vi "Sub Initialize.vi"(6 "Controller name":string, 8 "error in (no error)":errorcluster, 11 "Spectrum Recorder in":refnum<class "Spectrum Recorder too.lvclass">) -> (0 "error out":errorcluster, 2 "Initialize Result":refnum<class "Acquired Result.lvclass">, 3 "Spectrum Recorder out":refnum<class "Spectrum Recorder too.lvclass">)   [LabVIEW 2024, in "Spectrum Recorder too.lvclass"]
uses:
  Spectrum Recorder too.lvclass
  NHMFL_Core/Libraries/Instruments/Results/Acquired Result/Acquired Result.lvclass
  Worker/Worker Actor/Worker Actor.lvclass/Worker Actor.ctl
  Spectrum Recorder too.lvclass/Spectrum Recorder too.ctl
  Publish-Subscribe/Context.ctl
  <vilib>/ActorFramework/Actor/Actor.lvclass/Actor.ctl
  <vilib>/ActorFramework/Message Enqueuer/Message Enqueuer.lvclass/Message Enqueuer.ctl
  Publish-Subscribe/Interfaces/Publisher Messages/Subscribe Msg/Subscribe Msg.lvclass/Subscribe Msg.ctl
  NHMFL_Core/Libraries/Instruments/Instrument Driver/Worker State.ctl
  Write Fine region centers.vi
  Template Module/Write State.vi
  Template Module/Read State.vi
  <vilib>/ActorFramework/Message Enqueuer/Init from Existing Queue.vi
  <vilib>/ActorFramework/Message Enqueuer/Enqueue.vi
  Publish-Subscribe/Interfaces/Publisher Messages/Subscribe Msg/Subscribe Msg.lvclass
  Read Spectrum Recorder Configuration.vi
  <vilib>/ActorFramework/Message Priority Queue/Priority Enqueue.vi
  <vilib>/ActorFramework/Message Enqueuer/Message Enqueuer.lvclass
  Recorders/Continuous Recorder Actor/Continuous Recorder Actor.lvclass
  <vilib>/ActorFramework/Actor/Actor.lvclass
  D:/GitHub/LabActor/Recorders/Continuous Recorder Actor/Continuous Recorder Actor.lvclass
  D:/GitHub/LabActor/Instrument Actor/Instrument Actor.lvclass
  D:/GitHub/LabActor/Worker/Worker Actor/Worker Actor.lvclass
  D:/GitHub/LabActor/Template Module/Template Module.lvclass
  C:/Program Files/National Instruments/LabVIEW 2024/vi.lib/ActorFramework/Actor/Actor.lvclass
  D:/GitHub/LabActor/Worker/Woker Interface/Worker.lvclass
  D:/GitHub/LabActor/Recorders/Interfaces/Continuous Recorder/Continuous Recorder.lvclass
  D:/GitHub/LabActor/Spectrum Recorder too/Spectrum Recorder too.lvclass
  D:/GitHub/LabActor/Publish-Subscribe/Interfaces/Subscriber/Subscriber.lvclass
  NHMFL_Core/Libraries/Red Pitaya/RP Core/RP Transceiver/RP Transceiver.lvclass
  NHMFL_Core/Libraries/Red Pitaya/RP Core/RP Transceiver/Receiver format.ctl
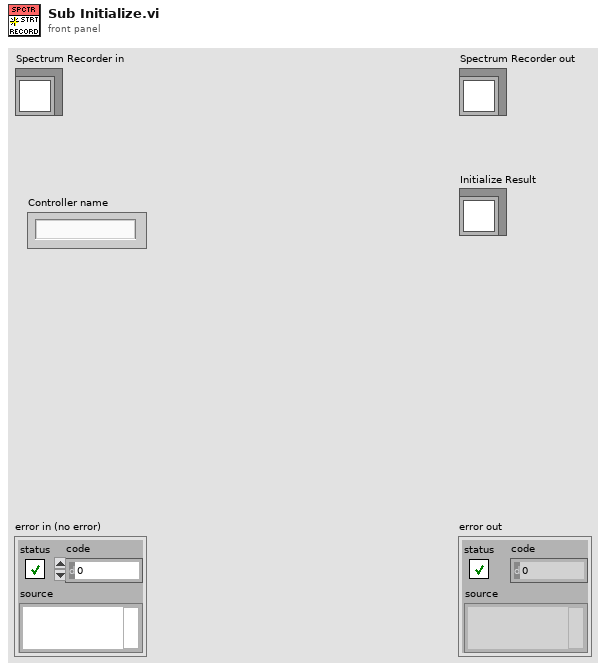
[diagram p1: front panel]
types:
  T1 = typedef "Receiver format.ctl" = enum16{"Hub 2xy", "Hub port 2xy 4f", "Hub ports 234", "X-Y-F", "F-X-Y", "X-Y", "X"}
  T2 = typedef "Context.ctl" = cluster{"Topic":string, "Source":string}
  T3 = typedef "Worker State.ctl" = enum16{"Idle", "Starting", "Working", "Stopping"}
  T4 = typedef "Spectrum Configuration.ctl" = cluster{"Start frequency":dbl, "End frequency":dbl, "Coarse step":dbl, "Step duration":dbl, "Red Pitaya address":string, "Open plot \non start":bool, "Regions width":dbl, "Fine step":dbl, "Pause between scans":dbl, "Clear rgs on start":bool, "Output amplitude":dbl, "Append measurements":string[], "Full scan period":dbl, "Full start":dbl, "Full end":dbl, "Full step":dbl}
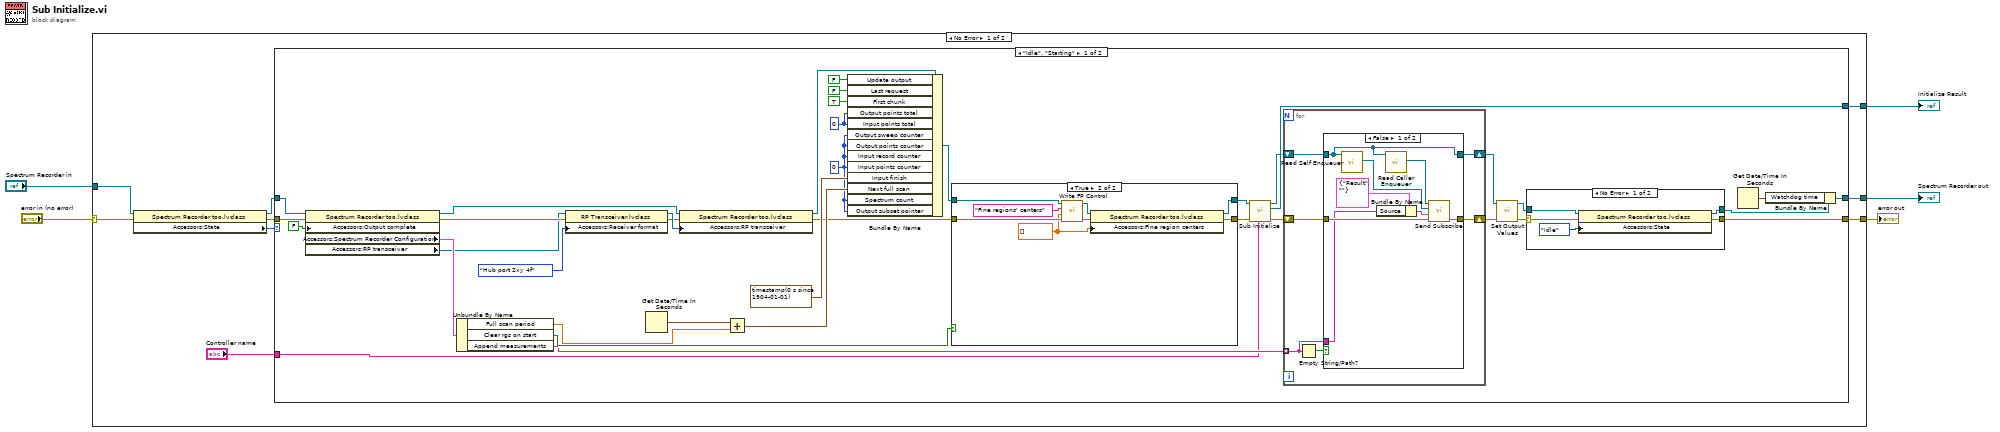
[diagram p0: block diagram]
diagram:
  n1 = case shown="No Error" "error in (no error)" {
    selector: "error in (no error)" -> [w9 w89]
    tunnel: [w12 w89] -> w4
    tunnel: [w14 w88] -> w2
    tunnel: "Spectrum Recorder in" -> [w13 w88]
    tunnel: [w7 _] -> w1
    frame No Error {
      n2 = property class="Spectrum Recorder too.lvclass"(reference=w13, error in=w9) -> (reference out=w11:refnum<class "Spectrum Recorder too.lvclass">, error out=w8:errorcluster, "Accessors:State"=w10:T3)
      n3 = case shown="\"Idle\", \"Starting\"" w10 {
        tunnel: w11 -> [w46 w87]
        tunnel: [w29 w87] -> w14
        tunnel: w8 -> [w45 w86]
        tunnel: [w52 w86] -> w12
        tunnel: [w43 _] -> w7
        tunnel: "Controller name" -> [w27 _]
        frame "Idle", "Starting" {
          w47 = i64 0 ("Output points total")
          w23 = 0 ("Output sweep counter")
          n4 = property class="Spectrum Recorder too.lvclass"(reference=w46, error in=w45, "Accessors:Output complete"=FALSE ("Output complete")) -> (reference out=w22:refnum<class "Spectrum Recorder too.lvclass">, error out=w20:errorcluster, "Accessors:Spectrum Recorder Configuration"=w40:T4, "Accessors:RP transceiver"=w19:refnum<class "RP Transceiver.lvclass">)
          n5 = Unbundle By Name(w40) -> ("Full scan period"=w25:dbl, "Clear rgs on start"=w39:bool, "Append measurements"=w34:string[])
          n6 = property class="RP Transceiver.lvclass"(reference=w19, error in=w20, "Accessors:Receiver format"=Receiver_format."Hub port 2xy 4f" ("Receiver format")) -> (reference out=w18:refnum<class "RP Transceiver.lvclass">, error out=w16:errorcluster)
          n7 = Get Date/Time In Seconds() -> (seconds since 1Jan1904=w26:timestamp)
          n8 = property class="Spectrum Recorder too.lvclass"(reference=w22, error in=w16, "Accessors:RP transceiver"=w18) -> (reference out=w17:refnum<class "Spectrum Recorder too.lvclass">, error out=w15:errorcluster)
          n9 = Add(x=w26, y=w25) -> (x+y=w24:timestamp)
          n10 = Bundle By Name(cluster=w17, "Update output"=FALSE, "Last request"=FALSE, "First chunk"=TRUE, "Output points total"=w47, "Input points total"=w47, "Output sweep counter"=w23, "Output points counter"=w23, "Input record counter"=w23, "Input points counter"=w23, "Input finish"=timestamp(0 s since 1904-01-01), "Next full scan"=w24, "Spectrum count"=w23, "Output subset pointer"=w23) -> (w38:refnum<class "Spectrum Recorder too.lvclass">)
          n11 = case shown="True" w39 {
            tunnel: w38 -> [w70 w78]
            tunnel: w15 -> [w69 w76]
            tunnel: [w69 w72] -> w37
            tunnel: [w70 w73] -> w36
            frame False {
            }
            frame True {
              w71 = dbl[] []
              n12 = call-dynamic "Write FP Control.vi"("error in (no error)"=w76, "Control Value"=w71, "Control Name"="Fine regions' centers", "Measure Object in"=w78) -> ("error out"=w74:errorcluster, "Measure Object out"=w75:refnum<class "Spectrum Recorder too.lvclass">)  [unwired: 6 in]
              n13 = property class="Spectrum Recorder too.lvclass"(reference=w75, error in=w74, "Accessors:Fine region centers"=w71) -> (reference out=w73:refnum<class "Spectrum Recorder too.lvclass">, error out=w72:errorcluster)
            }
          }
          n14 = call-parent "Sub Initialize.vi"("Controller name"=w27, "error in (no error)"=w37, "Instrument Recorder in"=w36) -> ("error out"=w32:errorcluster, "Initialize Result"=w43:refnum<class "Acquired Result.lvclass">, "Instrument Recorder out"=w33:refnum<class "Spectrum Recorder too.lvclass">)  [unwired: 6 in]
          n15 = for {
            tunnel: w34 -> [w55] mode=indexing
            shift-right: [w54] -> w31
            shift-left: w33 -> [w57]
            shift-right: [w53] -> w30
            shift-left: w32 -> [w56]
            n16 = Empty String/Path?(string/path=w55) -> (empty?=w58:bool)
            n17 = case shown="False" w58 {
              tunnel: w55 -> [w60 _]
              tunnel: w57 -> [w66 w68]
              tunnel: [w66 w68] -> w54
              tunnel: w56 -> [w65 w67]
              tunnel: [w59 w67] -> w53
              frame False {
                n18 = call <vilib>:"Read Self Enqueuer.vi"("Actor"=w66) -> ("Self Enqueuer"=w63:refnum<class "Message Enqueuer.lvclass">)  [unwired: 10 in]
                n19 = Bundle By Name(cluster=T2 {"Topic"="Result", "Source"=""} ("Context"), "Source"=w60) -> (w61:T2)
                n20 = call <vilib>:"Read Caller Enqueuer.vi"("Actor"=w66) -> ("Caller Enqueuer"=w64:refnum<class "Message Enqueuer.lvclass">)  [unwired: 10 in]
                n21 = call "Send Subscribe.vi"("error in (no error)"=w65, "Context"=w61, "Subscriber Enq"=w63, "Message Enqueuer"=w64) -> ("error out"=w59:errorcluster)  [unwired: 6 in, 1 out]
              }
              frame True {
              }
            }
          }
          n22 = call-dynamic "Set Output Values.vi"("error in (no error)"=w30, "Spectrum Recorder in"=w31) -> ("error out"=w50:errorcluster, "Spectrum Recorder out"=w49:refnum<class "Spectrum Recorder too.lvclass">)  [unwired: 8 in]
          n23 = case shown="No Error" w50 {
            selector: w50 -> [w83 w84]
            tunnel: [w80 w84] -> w52
            tunnel: w49 -> [w82 w85]
            tunnel: [w81 w85] -> w48
            frame No Error {
              n24 = property class="Spectrum Recorder too.lvclass"(reference=w82, error in=w83, "Accessors:State"=Worker_State."Idle" ("State")) -> (reference out=w81:refnum<class "Spectrum Recorder too.lvclass">, error out=w80:errorcluster)
            }
            frame Error {
            }
          }
          n25 = Get Date/Time In Seconds() -> (seconds since 1Jan1904=w28:timestamp)
          n26 = Bundle By Name(cluster=w48, "Watchdog time"=w28) -> (w29:refnum<class "Spectrum Recorder too.lvclass">)
        }
        frame "Working", Default {
        }
      }
    }
    frame Error {
    }
  }
  "error out" <- w4
  "Spectrum Recorder out" <- w2
  "Initialize Result" <- w1
